vi "ecg_wavelet.vi"() -> ()   [LabVIEW 2018]
uses:
  <vilib>/addons/Wavelet Analysis/application.llb/WA Detrend (Waveform).vi
  <vilib>/addons/Wavelet Analysis/online wavelet analysis.llb/WA Online Multiscale Peak Detection (Array).vi
  <vilib>/addons/_Advanced Signal Processing/NI_AdvSigProcWA.lvlib
  <vilib>/addons/_Advanced Signal Processing/NI_AdvSigProcOnlineWA.lvlib
panel:
  out "Waveform Graph 4":dynamicdata(graph)
  in  "Threshold frequency":dbl=0.0125 min=0.0 max=1.0 step=0.0001 format="%.4f"
  in  "Wavelet":u16(ring) items=["db02"=0, "db03"=1, "db04"=2, "db05"=3, "db06"=4, "db07"=5, "db08"=6, "db09"=7, "db10"=8, "db11"=9, "db12"=10, "db13"=11, "db14"=12, "Haar"=13, "bior1_3"=14, "bior1_5"=15, "bior2_2"=16, "bior2_4"=17, "bior2_6"=18, "bior2_8"=19, "bior3_1"=20, "bior3_3"=21, "bior3_5"=22, "bior3_7"=23, "bior3_9"=24, "bior4_4 (FBI)"=25, "bior5_5"=38, "bior6_8"=39, "coif1"=26, "coif2"=27, "coif3"=28, "coif4"=29, "coif5"=30, "sym2"=31, "sym3"=32, "sym4"=33, "sym5"=34, "sym6"=35, "sym7"=36, "sym8"=37]
  in  "Peak/Valley width 2":i32=32
  out "aspt-left-top":bool
  out "Peaks/Valleys Plot":cluster{"Ramp Pattern":dbl[], "X":dbl[]}[](graph)
  out "Waveform Graph 3":waveform(dbl)(graph)
  out "Waveform Graph 2":waveform(dbl)(graph)
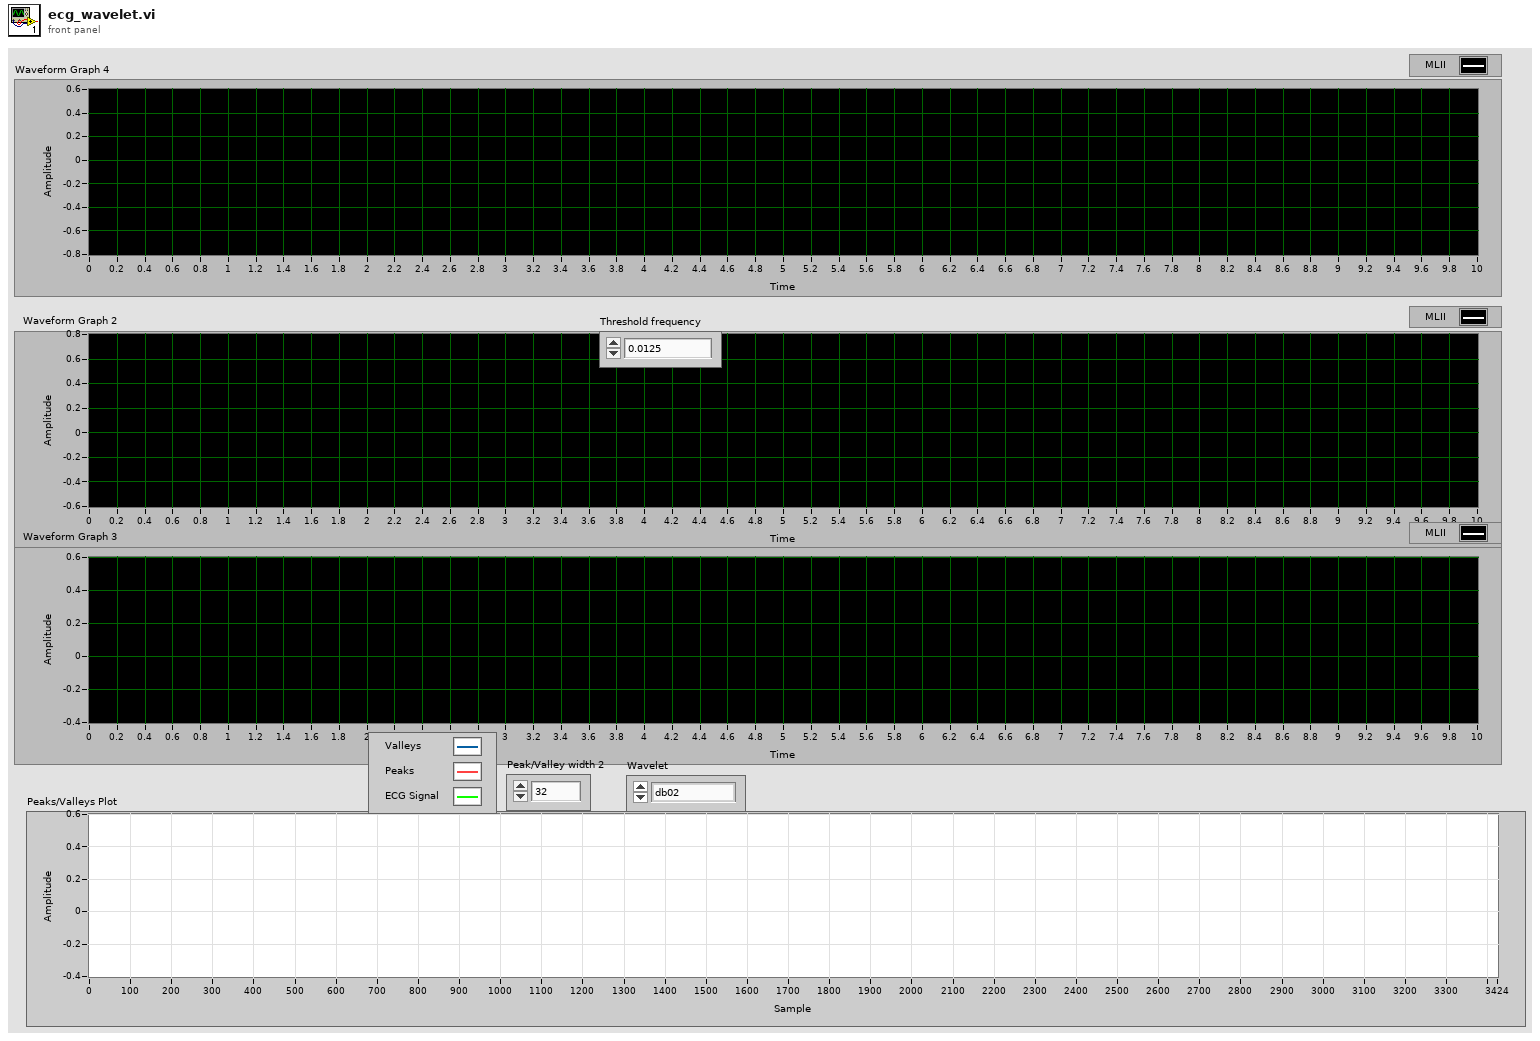
[diagram p1: front panel]
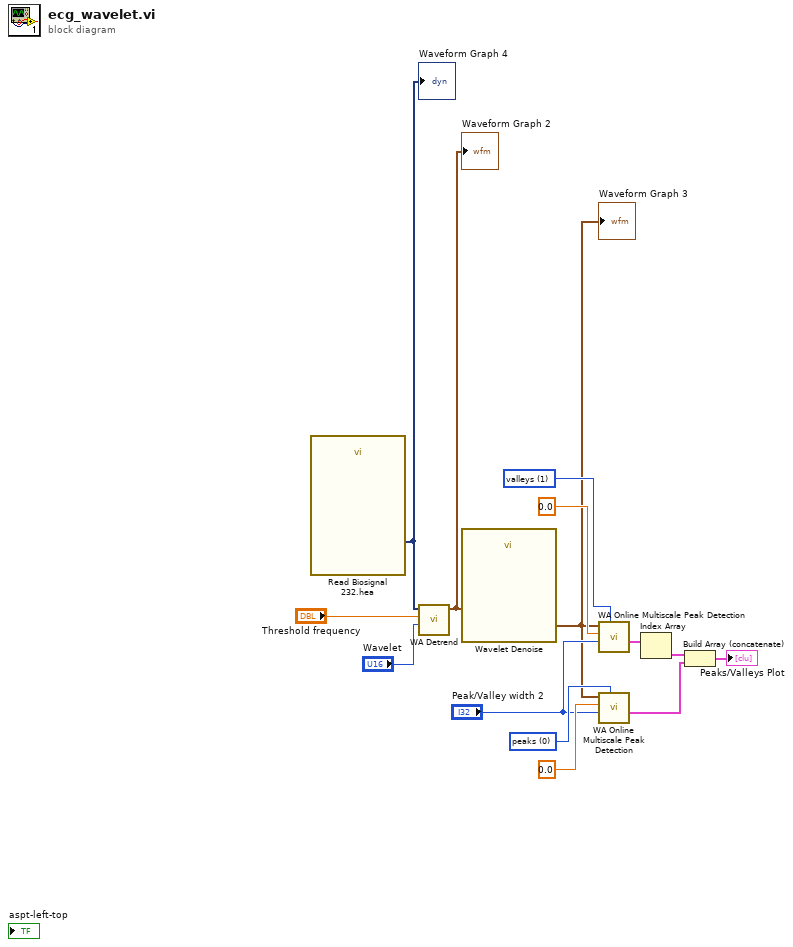
[diagram p0: block diagram]
diagram:
  w5 = u16 1 items=["peaks", "valleys"] ("peaks/valleys")
  w10 = u16 0 items=["peaks", "valleys"] ("peaks/valleys")
  n1 = call "Read Biosignal\n232.hea"() -> ("biosignals"=w3:dynamicdata)  [unwired: 11 in, 4 out]
  "Waveform Graph 4" <- w3
  n2 = call-poly <vilib>:"WA Detrend.vi"("wavelet"="Wavelet", "threshold frequency"="Threshold frequency", "signal"=w3) -> ("detrended signal"=w14:waveform(dbl))  [unwired: 6 in, 2 out]
  "Waveform Graph 2" <- w14
  n3 = call "Wavelet Denoise"("Signal"=w14) -> ("Denoised Signal"=w1:waveform(dbl))  [unwired: 9 in, 1 out]
  "Waveform Graph 3" <- w1
  n4 = call-poly <vilib>:"WA Online Multiscale Peak Detection.vi"("peaks/valleys"=w5, "width"="Peak/Valley width 2", "threshold"=0.0 ("Threshold"), "signal"=w1) -> ("peak plot"=w7:cluster{"Ramp Pattern":dbl[], "X":dbl[]}[])  [unwired: 4 in, 3 out]
  n5 = call-poly <vilib>:"WA Online Multiscale Peak Detection.vi"("peaks/valleys"=w10, "width"="Peak/Valley width 2", "threshold"=0.0 ("Threshold"), "signal"=w1) -> ("peak plot"=w13:cluster{"Ramp Pattern":dbl[], "X":dbl[]}[])  [unwired: 4 in, 3 out]
  n6 = Index Array(array=w7) -> (element=w12:cluster{"Ramp Pattern":dbl[], "X":dbl[]})  [unwired: 1 in]
  n7 = Build Array (concatenate)(w12, w13) -> (→"Peaks/Valleys Plot":cluster{"Ramp Pattern":dbl[], "X":dbl[]}[])
